vi "FMA1600A General Setup.vi"(5 "Gas Type":T4, 6 "Skip Dialog":bool, 7 "Unit ID":string, 8 "error in (no error)":errorcluster, 9 "Select Gas?":bool=TRUE, 10 "Set STP Register":bool, 11 "VISA Refnum in":refnum<visa-resource-name>) -> (0 "error out":errorcluster, 1 "Data Frame Format":T1, 2 "Measurement Units":T2, 3 "VISA Refnum out":refnum<visa-resource-name>)   [LabVIEW 2020]
uses:
  Type Definitions/FMA1600A Gas Type.ctl
  Type Definitions/FMA1600A Units String.ctl
  Units of Measure.ctl
  Data Frame.ctl
  Type Definitions/FMA1600A Commands.ctl
  <vilib>/Utility/error.llb/whitespace.ctl
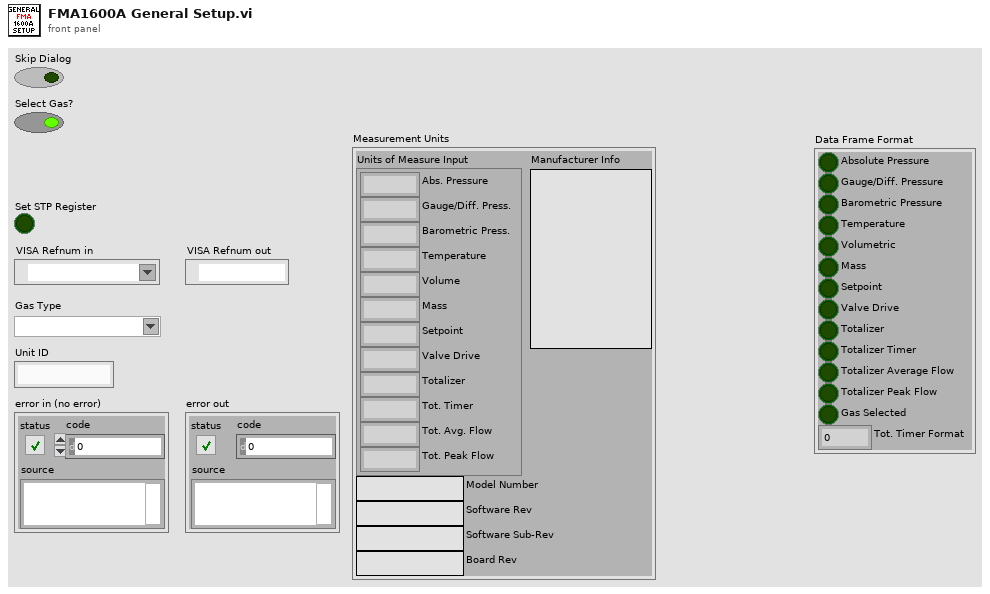
[diagram p1: front panel]
types:
  T1 = typedef "Data Frame.ctl" = cluster{"Absolute Pressure":bool, "Gauge/Diff. Pressure":bool, "Barometric Pressure":bool, "Temperature":bool, "Volumetric":bool, "Mass":bool, "Setpoint":bool, "Valve Drive":bool, "Totalizer":bool, "Totalizer Timer":bool, "Totalizer Average Flow":bool, "Totalizer Peak Flow":bool, "Gas Selected":bool, "Tot. Timer Format":u16}
  T2 = typedef "FMA1600A Units String.ctl" = cluster{"Software Rev":string, "Model Number":string, "Manufacturer Info":string, "Software Sub-Rev":string, "Board Rev":string, "Units of Measure Input":T3}
  T3 = typedef "Units of Measure.ctl" = cluster{"Abs. Pressure":string, "Gauge/Diff. Press.":string, "Barometric Press.":string, "Temperature":string, "Volume":string, "Mass":string, "Setpoint":string, "Valve Drive":string, "Totalizer":string, "Tot. Timer":string, "Tot. Avg. Flow":string, "Tot. Peak Flow":string}
  T4 = typedef "FMA1600A Gas Type.ctl" = string
  T5 = enum8{"2400", "9600", "19200", "38400", "57600", "115200", "Unknown"}
  T6 = cluster{"Valve Drive":bool, "Totalizer":bool, "Totalizer Timer":bool, "Totalizer Peak Flow":bool, "Show Abs., Gauge\nand Baro. pressures":bool}
  T7 = cluster{"Pressure(s)":bool, "Temperature":bool, "Volumetric":bool, "Mass":bool, "Totalizer Average Flow":bool, "Gas Selected":bool}
  T8 = typedef "whitespace.ctl" = u16
  T9 = typedef "FMA1600A Commands.ctl" = string
  T10 = cluster{"Unit ID":string, "Baud Rate":enum8{"2400", "9600", "19200", "38400", "57600", "115200", "Unknown"}, "VISA Sesssion In":refnum<visa-resource-name>}
  T11 = cluster{"Abs. Pressure":string, "Gauge/Diff. Press.":string, "Barometric Press.":string, "Temperature":string, "Volume":string, "Mass":string, "Setpoint":string, "Valve Drive":string, "Totalizer":string, "Tot. Timer":string, "Tot. Avg. Flow":string, "Tot. Peak Flow":string}
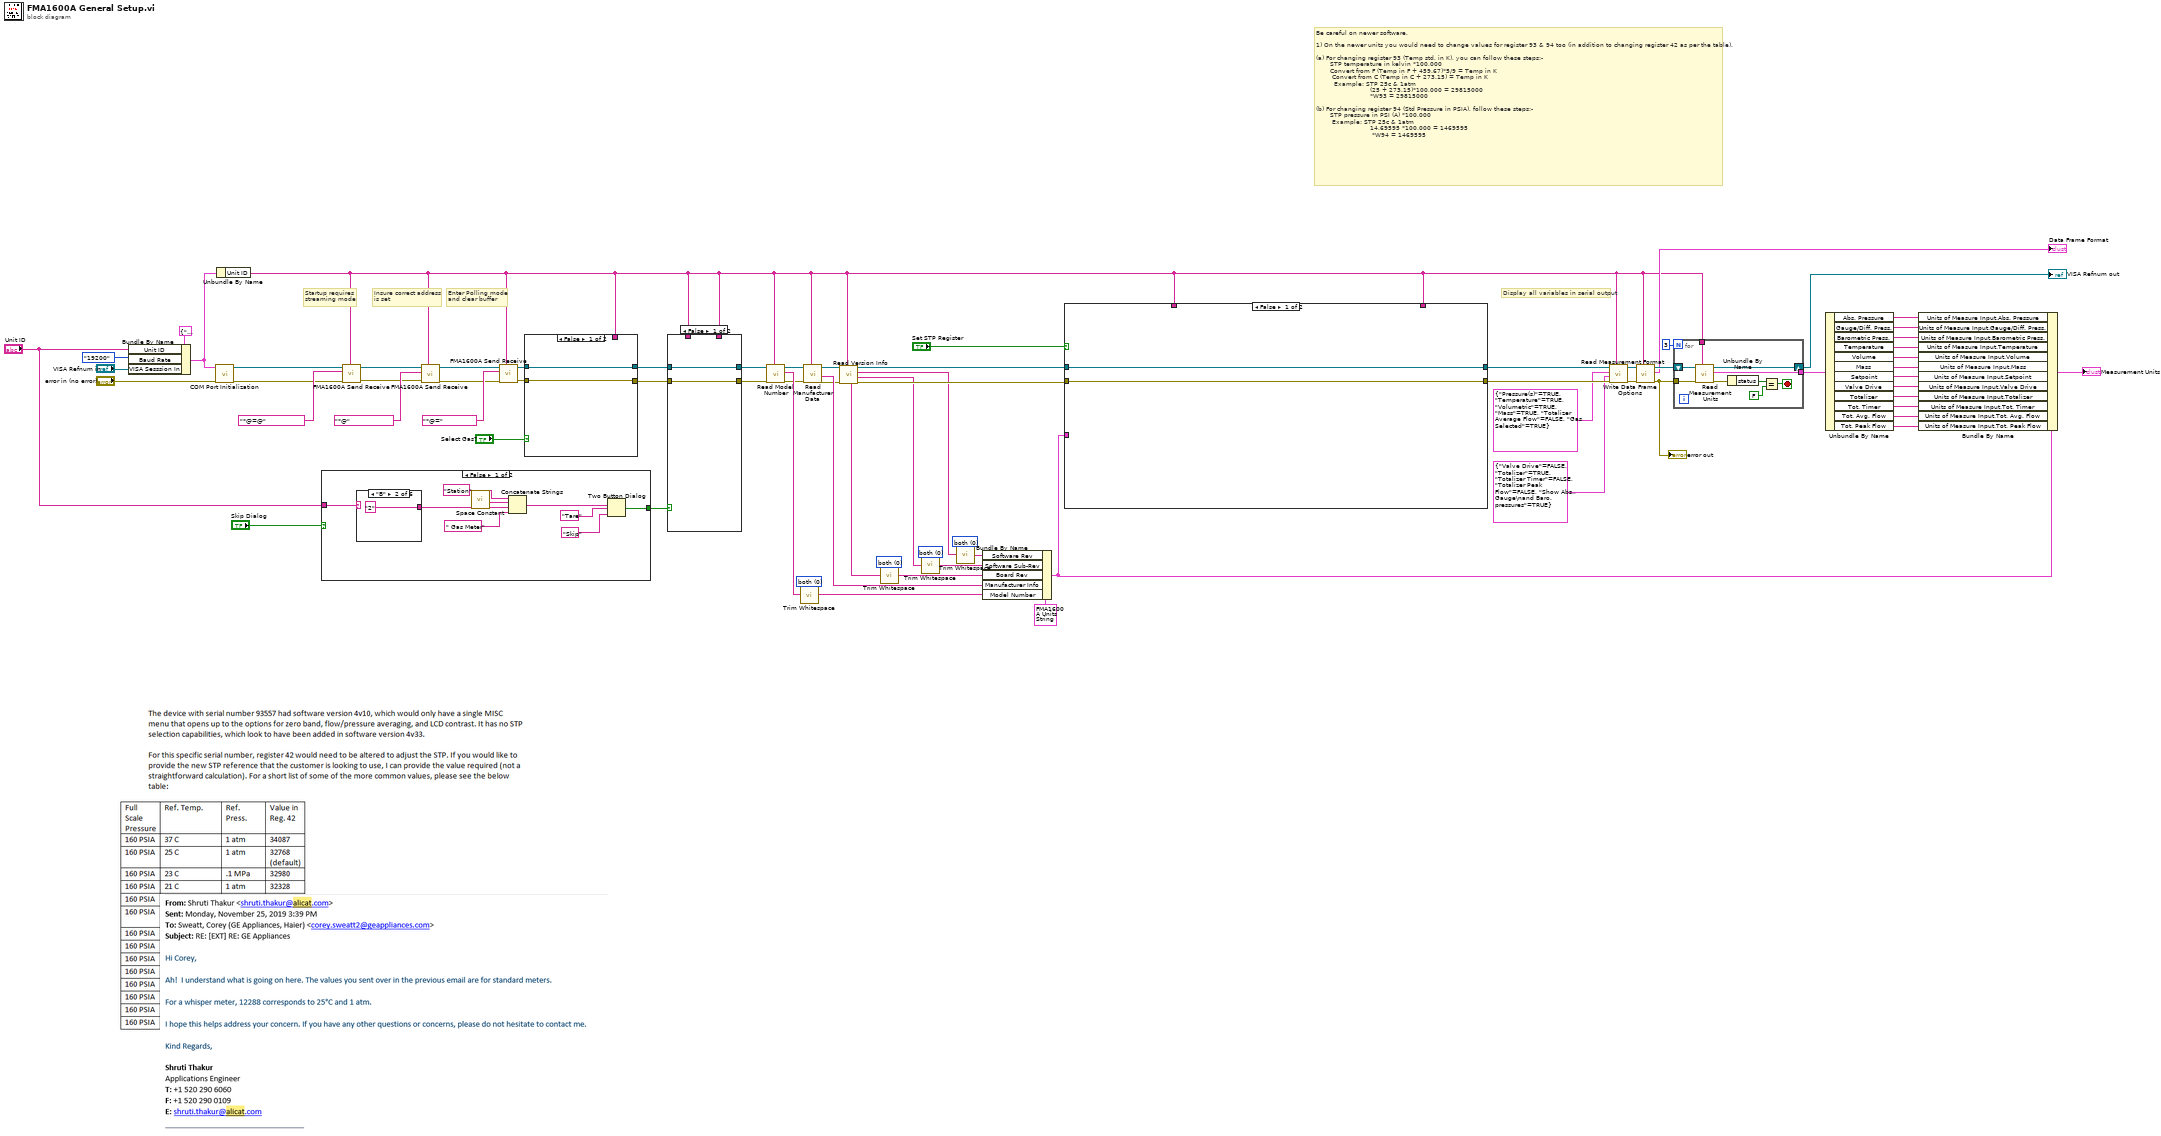
[diagram p0: block diagram]
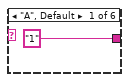
[diagram p2: hidden frame]
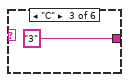
[diagram p3: hidden frame]
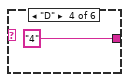
[diagram p4: hidden frame]
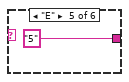
[diagram p5: hidden frame]
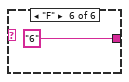
[diagram p6: hidden frame]
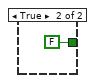
[diagram p7: hidden frame]
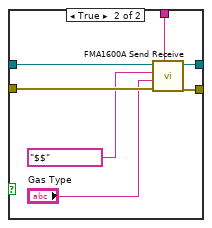
[diagram p8: hidden frame]
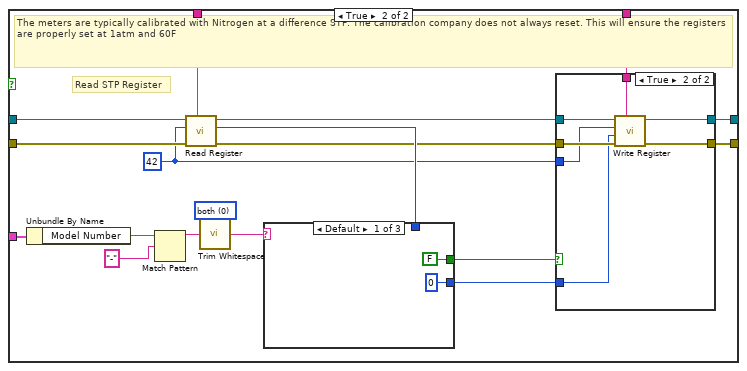
[diagram p9: hidden frame]
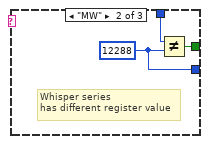
[diagram p11: hidden frame]
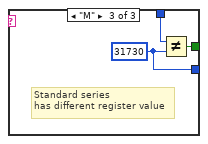
[diagram p12: hidden frame]
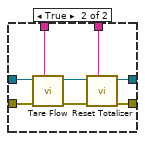
[diagram p13: hidden frame]
diagram:
  w18 = T8 0 items=["both", "start of string", "end of string"] ("location (both)")
  w19 = T8 0 items=["both", "start of string", "end of string"] ("location (both)")
  w22 = T8 0 items=["both", "start of string", "end of string"] ("location (both)")
  w23 = T8 0 items=["both", "start of string", "end of string"] ("location (both)")
  # "Display all variables in serial output"
  # "Enter Polling mode\nand clear buffer"
  # "Startup requires \nstreaming mode"
  # "Insure correct address\nis set"
  # "Be careful on newer software.\n\n1) On the newer units you would need to change values for register 93 & 94 too (in addition to changing register 42 as per the table). \n\n(a) For changing register 93 (Temp std. in K), you can follow these steps:-\n       STP temperature in kelvin *100,000\n       Convert from F (Temp in F + 459.67)*5/9 = Temp in K\n        Convert from C (Temp in C + 273.15) = Temp in K\n         Example: STP 25c & 1atm\n                           (25 + 273.15)*100,000 = 29815000\n                           *W93 = 29815000\n\n(b) For changing register 94 (Std Pressure in PSIA), follow these steps:-\n       STP pressure in PSI (A) *100,000\n        Example: STP 25c & 1atm\n                           14.69595 *100,000 = 1469595\n                            *W94 = 1469595"
  n1 = Bundle By Name(cluster=T10 {"Unit ID"="A", "Baud Rate"=enum."19200", "VISA Sesssion In"="COM1"} ("Communication Settings"), "Unit ID"="Unit ID", "Baud Rate"=T5."19200", "VISA Sesssion In"="VISA Refnum in") -> (w63:T10)
  n2 = call "COM Port Initialization.vi"("error in (no error)"="error in (no error)", "Communication Settings"=w63) -> ("error out"=w60:errorcluster, "VISA Session Out"=w59:refnum<visa-resource-name>)  [unwired: 8 in]
  n3 = Unbundle By Name(w63) -> ("Unit ID"=w9:string)
  n4 = case shown="False" "Skip Dialog" {
    tunnel: [w81 FALSE ("T button?")] -> w72
    tunnel: "Unit ID" -> [w73 _]
    frame False {
      n5 = case shown="\"B\"" w73 {
        tunnel: ["1" ("message") "2" ("message") "3" ("message") "4" ("message") "5" ("message") "6" ("message")] -> w79
        frame "A", Default {
        }
        frame "B" {
        }
        frame "C" {
        }
        frame "D" {
        }
        frame "E" {
        }
        frame "F" {
        }
      }
      n6 = call <vilib>:"Space Constant.vi"() -> ("String"=w74:string)
      n7 = Concatenate Strings("Station" ("message"), w74, w79, " Gas Meter" ("string")) -> (w76:string)
      n8 = Two Button Dialog(message=w76, 1:"Skip" ("F button name (\"Cancel\")"), 2:"Tare" ("T button name (\"OK\")")) -> (T button?=w81:bool)
    }
    frame True {
    }
  }
  n9 = call "FMA1600A Send Receive.vi"("Unit ID"=w9, "error in (no error)"=w60, "FMA1600A Commands"=T9 "*@=@", "VISA Refnum in"=w59) -> ("error out"=w58:errorcluster, "VISA Refnum out"=w57:refnum<visa-resource-name>)  [unwired: 5 in, 1 out]
  n10 = call "FMA1600A Send Receive.vi"("Unit ID"=w9, "error in (no error)"=w58, "FMA1600A Commands"=T9 "*@", "VISA Refnum in"=w57) -> ("error out"=w52:errorcluster, "VISA Refnum out"=w53:refnum<visa-resource-name>)  [unwired: 5 in, 1 out]
  n11 = call "FMA1600A Send Receive.vi"("Unit ID"=w9, "error in (no error)"=w52, "FMA1600A Commands"=T9 "*@=", "VISA Refnum in"=w53) -> ("error out"=w56:errorcluster, "VISA Refnum out"=w55:refnum<visa-resource-name>)  [unwired: 5 in, 1 out]
  n12 = case shown="False" "Select Gas?" {
    tunnel: w56 -> [w90 w97]
    tunnel: w55 -> [w89 w96]
    tunnel: [w89 w93] -> w51
    tunnel: [w90 w92] -> w50
    tunnel: w9 -> [_ w91]
    frame False {
    }
    frame True {
      n13 = call "FMA1600A Send Receive.vi"("Unit ID"=w91, "error in (no error)"=w97, "Gas Type"="Gas Type", "FMA1600A Commands"=T9 "$$", "VISA Refnum in"=w96) -> ("error out"=w92:errorcluster, "VISA Refnum out"=w93:refnum<visa-resource-name>)  [unwired: 4 in, 1 out]
    }
  }
  n14 = case shown="False" w72 {
    tunnel: [w98 w100] -> w34
    tunnel: [w99 w101] -> w35
    tunnel: w50 -> [w99 w106]
    tunnel: w51 -> [w98 w105]
    tunnel: w9 -> [_ w107]
    tunnel: w9 -> [_ w102]
    frame False {
    }
    frame True {
      n15 = call "Tare Flow.vi"("Unit ID (A)"=w107, "error in"=w106, "VISA Session In"=w105) -> ("error out"=w104:errorcluster, "VISA Session Out"=w103:refnum<visa-resource-name>)  [unwired: 7 in]
      n16 = call "Reset Totalizer.vi"("Unit ID (A)"=w102, "error in"=w104, "VISA Session In"=w103) -> ("error out"=w101:errorcluster, "VISA Session Out"=w100:refnum<visa-resource-name>)  [unwired: 6 in, 1 out]
    }
  }
  n17 = call "Read Model Number.vi"("Unit ID (A)"=w9, "error in"=w35, "VISA Session In"=w34) -> ("error out"=w5:errorcluster, "Model Number"=w25:string, "VISA Session Out"=w4:refnum<visa-resource-name>)  [unwired: 6 in]
  n18 = call <vilib>:"Trim Whitespace.vi"("string"=w25, "location (both)"=w23) -> ("trimmed string"=w24:string)
  n19 = call "Read Manufacturer Data.vi"("Unit ID (A)"=w9, "error in"=w5, "VISA Session In"=w4) -> ("error out"=w2:errorcluster, "Manufacturer Info"=w30:string, "VISA Session Out"=w3:refnum<visa-resource-name>)  [unwired: 6 in]
  n20 = call "Read Version Info.vi"("Unit ID (A)"=w9, "error in"=w2, "VISA Session In"=w3) -> ("error out"=w33:errorcluster, "Software Sub-Rev"=w17:string, "Software Rev"=w21:string, "VISA Session Out"=w32:refnum<visa-resource-name>, "Board Rev"=w15:string)  [unwired: 4 in]
  n21 = call <vilib>:"Trim Whitespace.vi"("string"=w15, "location (both)"=w19) -> ("trimmed string"=w14:string)
  n22 = call <vilib>:"Trim Whitespace.vi"("string"=w17, "location (both)"=w18) -> ("trimmed string"=w16:string)
  n23 = call <vilib>:"Trim Whitespace.vi"("string"=w21, "location (both)"=w22) -> ("trimmed string"=w20:string)
  n24 = Bundle By Name(cluster=T2 {"Software Rev"="", "Model Number"="", "Manufacturer Info"="", "Software Sub-Rev"="", "Board Rev"="", "Units of Measure Input"={"Abs. Pressure"="", "Gauge/Diff. Press."="", "Barometric Press."="", "Temperature"="", "Volume"="", "Mass"="", "Setpoint"="", "Valve Drive"="", "Totalizer"="", "Tot. Timer"="", "Tot. Avg. Flow"="", "Tot. Peak Flow"=""}} ("Measurement Units"), "Software Rev"=w20, "Software Sub-Rev"=w16, "Board Rev"=w14, "Manufacturer Info"=w30, "Model Number"=w24) -> (w29:T2)
  n25 = case shown="False" "Set STP Register" {
    tunnel: [w108 w114] -> w11
    tunnel: [w109 w117] -> w13
    tunnel: w33 -> [w109 w126]
    tunnel: w32 -> [w108 w127]
    tunnel: w9 -> [_ w110]
    tunnel: w9 -> [_ w116]
    tunnel: w29 -> [_ w125]
    frame False {
    }
    frame True {
      w121 = T8 0 items=["both", "start of string", "end of string"] ("location (both)")
      w113 = u16 42 ("Register address")
      # "Read STP Register"
      # "The meters are typically calibrated with Nitrogen at a difference STP. The calibration company does not always reset. This will ensure the registers are properly set at 1atm and 60F"
      n26 = Unbundle By Name(w125) -> ("Model Number"=w124:string)
      n27 = Match Pattern(string=w124, regular expression="-" ("search string")) -> (before substring=w122:string)  [unwired: 1 in, 3 out]
      n28 = call "Read Register.vi"("Unit ID (A)"=w110, "error in"=w126, "Register address"=w113, "VISA Session In"=w127) -> ("error out"=w118:errorcluster, "Register Value (I32)"=w119:i32, "VISA Session Out"=w115:refnum<visa-resource-name>)  [unwired: 5 in]
      n29 = call <vilib>:"Trim Whitespace.vi"("string"=w122, "location (both)"=w121) -> ("trimmed string"=w120:string)
      n30 = case shown="Default" w120 {
        tunnel: w119 -> [_ w141 w144]
        tunnel: [FALSE w140 w143] -> w111
        tunnel: [0 ("y") w139 w142] -> w112
        frame Default {
        }
        frame "MW" {
          w139 = 12288 ("y")
          # "Whisper series\nhas different register value"
          n31 = Not Equal?(x=w141, y=w139) -> (x != y?=w140:bool)
        }
        frame "M" {
          w142 = 31730 ("y")
          # "Standard series\nhas different register value"
          n32 = Not Equal?(x=w144, y=w142) -> (x != y?=w143:bool)
        }
      }
      n33 = case shown="True" w111 {
        tunnel: w118 -> [w129 w136]
        tunnel: [w129 w135] -> w117
        tunnel: w116 -> [_ w134]
        tunnel: w115 -> [w128 w133]
        tunnel: [w128 w132] -> w114
        tunnel: w113 -> [_ w131]
        tunnel: w112 -> [_ w130]
        frame False {
        }
        frame True {
          n34 = call "Write Register.vi"("Unit ID (A)"=w134, "error in"=w136, "Register Value"=w130, "Register address"=w131, "VISA Session In"=w133) -> ("error out"=w135:errorcluster, "VISA Session Out"=w132:refnum<visa-resource-name>)  [unwired: 4 in, 1 out]
        }
      }
    }
  }
  n35 = call "Write Data Frame Options.vi"("Unit ID (A)"=w9, "error in"=w13, "Enables: Data frame only"=T6 {"Valve Drive"=FALSE, "Totalizer"=TRUE, "Totalizer Timer"=FALSE, "Totalizer Peak Flow"=FALSE, "Show Abs., Gauge\nand Baro. pressures"=TRUE}, "Enables: \nData frame and Display"=T7 {"Pressure(s)"=TRUE, "Temperature"=TRUE, "Volumetric"=TRUE, "Mass"=TRUE, "Totalizer Average Flow"=FALSE, "Gas Selected"=TRUE} ("Enables: \nData frame and Display"), "VISA Session In"=w11) -> ("error out"=w12:errorcluster, "VISA Session Out"=w10:refnum<visa-resource-name>)  [unwired: 5 in]
  n36 = call "Read Measurement Format.vi"("Unit ID (A)"=w9, "error in"=w12, "VISA Session In"=w10) -> ("error out"=w26:errorcluster, "Data Frame Format"=→"Data Frame Format":T1, "VISA Session Out"=w28:refnum<visa-resource-name>)  [unwired: 6 in]
  "error out" <- w26
  n37 = for {
    N: 3 -> [_]
    tunnel: w9 -> [w147]
    tunnel: [w149] -> w49
    shift-right: [w150] -> w70
    shift-left: w28 -> [w151]
    tunnel: w26 -> [w148]
    stop <- w152 stop-if-true
    n38 = call "Read Measurement Units.vi"("Unit ID (A)"=w147, "error in"=w148, "VISA Session In"=w151) -> ("error out"=w153:errorcluster, "Measurement Units"=w149:T11, "VISA Session Out"=w150:refnum<visa-resource-name>)  [unwired: 5 in, 1 out]
    n39 = Unbundle By Name(w153) -> ("status"=w146:bool)
    n40 = Equal?(x=w146, y=FALSE ("x")) -> (x = y?=w152:bool)
  }
  "VISA Refnum out" <- w70
  n41 = Unbundle By Name(w49) -> ("Abs. Pressure"=w47:string, "Gauge/Diff. Press."=w46:string, "Barometric Press."=w45:string, "Temperature"=w44:string, "Volume"=w43:string, "Mass"=w42:string, "Setpoint"=w41:string, "Valve Drive"=w40:string, "Totalizer"=w39:string, "Tot. Timer"=w38:string, "Tot. Avg. Flow"=w37:string, "Tot. Peak Flow"=w36:string)
  n42 = Bundle By Name(cluster=w29, "Units of Measure Input.Abs. Pressure"=w47, "Units of Measure Input.Gauge/Diff. Press."=w46, "Units of Measure Input.Barometric Press."=w45, "Units of Measure Input.Temperature"=w44, "Units of Measure Input.Volume"=w43, "Units of Measure Input.Mass"=w42, "Units of Measure Input.Setpoint"=w41, "Units of Measure Input.Valve Drive"=w40, "Units of Measure Input.Totalizer"=w39, "Units of Measure Input.Tot. Timer"=w38, "Units of Measure Input.Tot. Avg. Flow"=w37, "Units of Measure Input.Tot. Peak Flow"=w36) -> (→"Measurement Units":T2)
